vi "DrawSingleRGBCurve.vi"(3 "color( default is black)":u32, 4 "Point Position Cluster Array":cluster{i16, i16}[](array[cluster]), 5 "picture to be draw curve":picture) -> (2 "new picture":picture)   [LabVIEW 2016]
panel:
  # "This VI is to draw a cure by Turn point position orderly"
  # "Turn point 's  postion(x,y)  of curve"
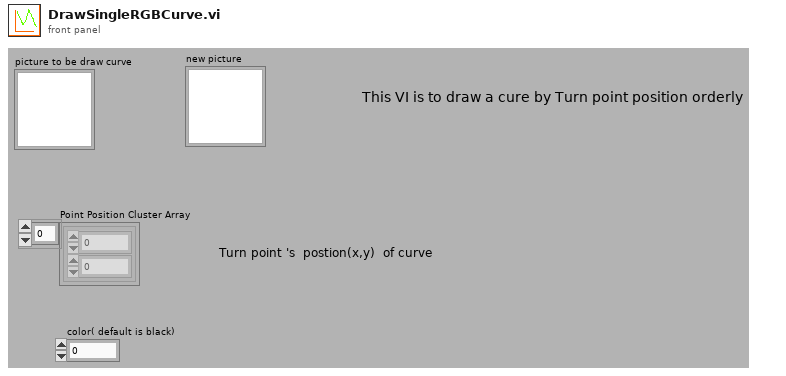
[diagram p1: front panel]
types:
  T1 = cluster{"Width":u16, "Style":enum32{"Solid", "Dash", "Dot", "DashDot", "DashDotDot"}}
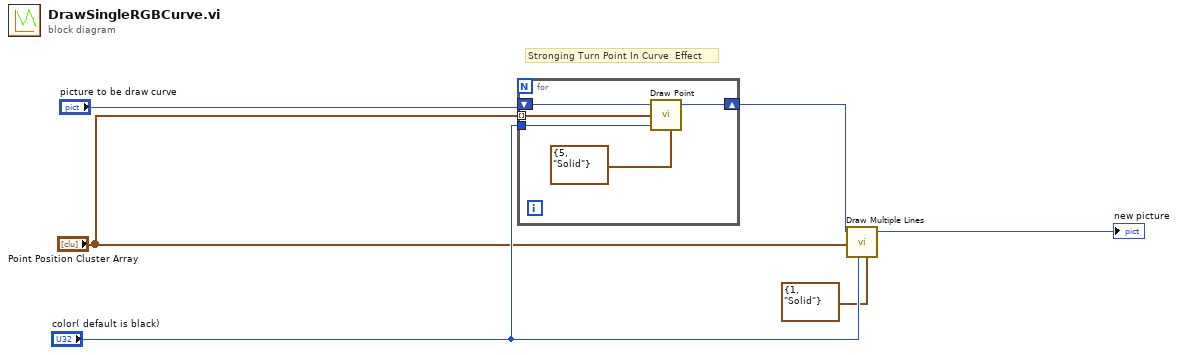
[diagram p0: block diagram]
diagram:
  # "Stronging Turn Point In Curve  Effect"
  n1 = for {
    tunnel: "Point Position Cluster Array" -> [w11] mode=indexing
    shift-right: [w10] -> w4
    shift-left: "picture to be draw curve" -> [w9]
    tunnel: "color( default is black)" -> [w7]
    n2 = call <vilib>:"Draw Point.vi"("picture"=w9, "point(x,y)"=w11, "color(black)"=w7, "pen"=T1 {"Width"=5, "Style"=enum."Solid"}) -> ("new picture"=w10:picture)  [unwired: 5 out]
  }
  n3 = call <vilib>:"Draw Multiple Lines.vi"("picture"=w4, "line endpoints"="Point Position Cluster Array", "color(black)"="color( default is black)", "pen"=T1 {"Width"=1, "Style"=enum."Solid"}) -> ("new picture"=→"new picture":picture)  [unwired: 1 in, 4 out]
